vi "数据库更新.vi"(0 "设备号":string(combo)="01", 9 "数据":string[](array[string])=["123456", "ZHANG", "1", "1", "20150718", "20150719", "5", "Q14073-01", "100", "100", "100", "100", "200", "200", "200", "300", "300", "300", "300", "300", "300", "300", "300"], 11 "error in (no error)":errorcluster) -> (15 "error out":errorcluster)   [LabVIEW 2013]
panel:
  out "连接的字符串":string
  in  "数据名":string[](array[string])=["CZZ", "WC", "HG", "KSSJ", "JSSJ", "FGCS", "SBID", "Date1", "Date2", "Date3", "Date4", "Date5", "Date6", "Date7", "Date8", "Date9", "Date10", "Date11", "Date12", "Date13", "Date14", "Date15"]
  # "CZZ\nWC\nHG\nKSSJ\nJSSJ\nFGCS\nSBID\nDate1\nDate2\nDate3\nDate4\nDate5\nDate6\nDate7\nDate8\nDate9\nDate10\nDate11\nDate12\nDate13\nDate14\nDate15"
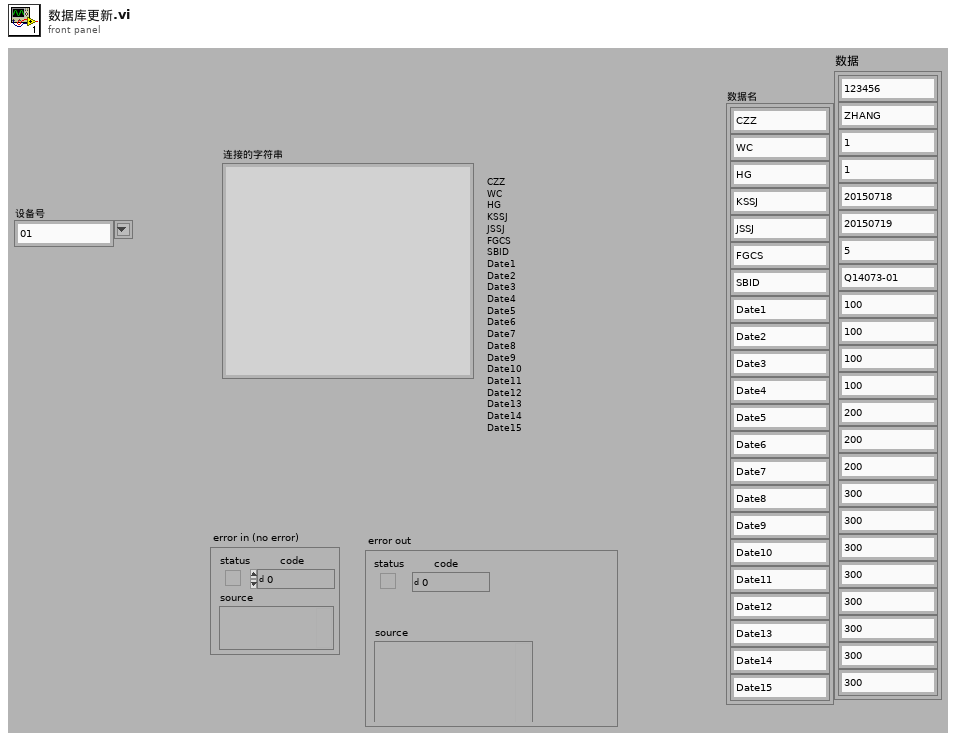
[diagram p1: front panel]
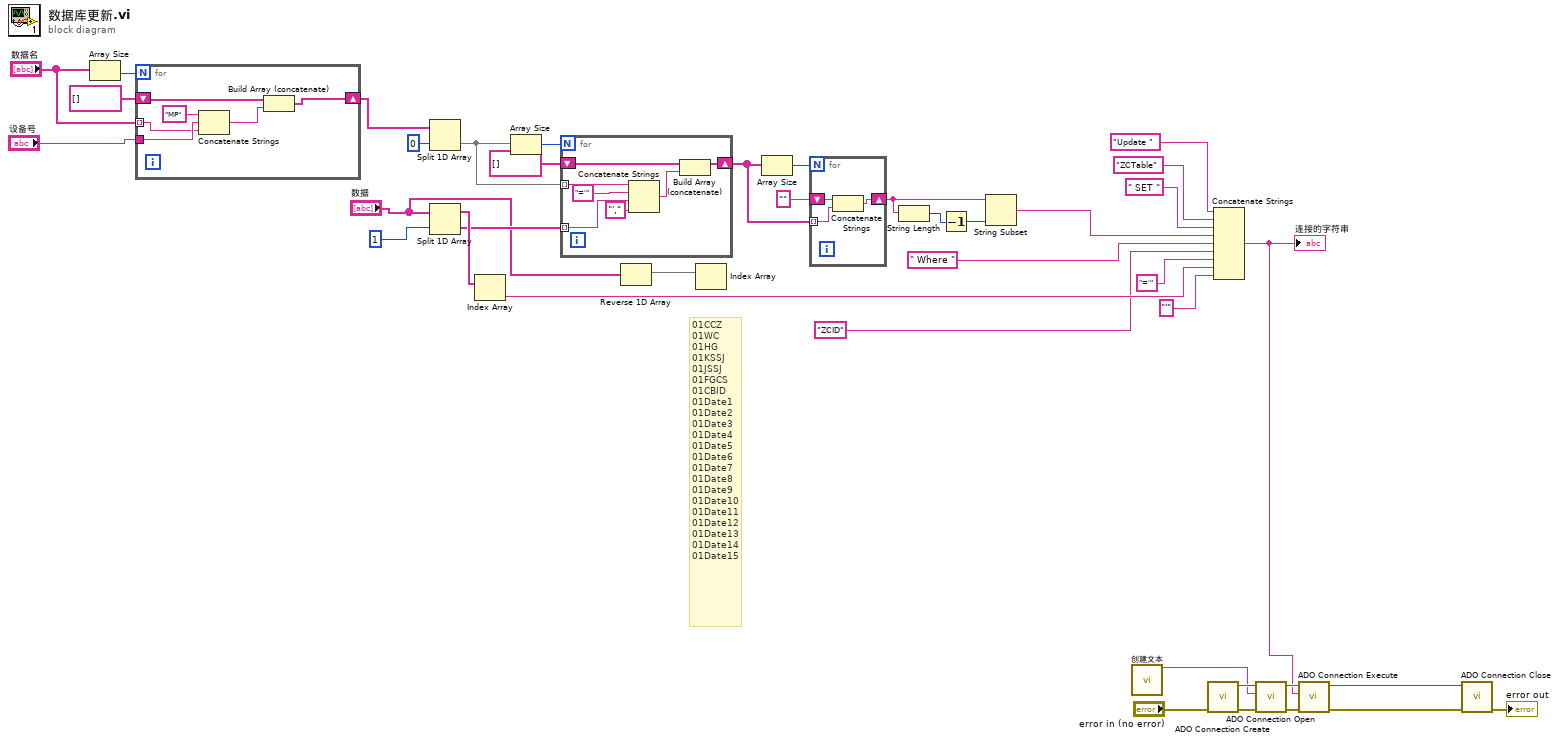
[diagram p0: block diagram]
diagram:
  # "01CCZ\n01WC\n01HG\n01KSSJ\n01JSSJ\n01FGCS\n01CBID\n01Date1\n01Date2\n01Date3\n01Date4\n01Date5\n01Date6\n01Date7\n01Date8\n01Date9\n01Date10\n01Date11\n01Date12\n01Date13\n01Date14\n01Date15"
  n1 = Array Size(array="数据名") -> (size(s)=w11:i32)
  n2 = for {
    N: w11 -> [_]
    tunnel: "数据名" -> [w41] mode=indexing
    shift-right: [w43] -> w7
    shift-left: string[] [] -> [w45]
    tunnel: "设备号" -> [w42]
    n3 = Concatenate Strings("MP" ("字符串"), w42, w41) -> (w44:string)
    n4 = Build Array (concatenate)(w45, w44) -> (w43:string[])
  }
  n5 = Split 1D Array(array=w7, index=0 ("索引")) -> (second subarray=w27:string[])  [unwired: 1 out]
  n6 = Split 1D Array(array="数据", index=1 ("索引列")) -> (first subarray=w29:string[], second subarray=w26:string[])
  n7 = Index Array(array=w29) -> (element=w14:string)  [unwired: 1 in]
  n8 = Array Size(array=w27) -> (size(s)=w28:i32)
  n9 = for {
    N: w28 -> [_]
    tunnel: w27 -> [w52] mode=indexing
    shift-right: [w49] -> w24
    shift-left: string[] [] -> [w48]
    tunnel: w26 -> [w47] mode=indexing
    n10 = Concatenate Strings(w52, "='" ("字符串"), w47, "'," ("字符串")) -> (w50:string)
    n11 = Build Array (concatenate)(w48, w50) -> (w49:string[])
  }
  n12 = Reverse 1D Array(array="数据") -> (reversed array=w6:string[])
  n13 = Index Array(array=w6) -> ()  [unwired: 1 in, 1 out]
  n14 = Array Size(array=w24) -> (size(s)=w25:i32)
  n15 = for {
    N: w25 -> [_]
    tunnel: w24 -> [w55] mode=indexing
    shift-right: [w54] -> w23
    shift-left: "" -> [w53]
    n16 = Concatenate Strings(w53, w55) -> (w54:string)
  }
  n17 = String Length(string=w23) -> (length=w4:i32)
  n18 = Decrement(x=w4) -> (x-1=w3:i32)
  n19 = String Subset(string=w23, length (rest)=w3) -> (substring=w2:string)  [unwired: 1 in]
  n20 = call "创建文本"() -> ("Result"=w31:string)  [unwired: 14 in, 1 out]
  n21 = call "ADO Connection Create.vi"("error in (no error)"="error in (no error)") -> ("error out"=w38:errorcluster, "ADODB._Connection Out"=w37:refnum<k7>)  [unwired: 9 out]
  n22 = Concatenate Strings("Update " ("字符串"), "ZCTable" ("数据库名"), " SET " ("字符串"), w2, " Where " ("字符串"), "ZCID" ("索引列名"), "='" ("字符串"), w14, "'" ("字符串")) -> (w5:string)
  "连接的字符串" <- w5
  n23 = call "ADO Connection Open.vi"("error in (no error)"=w38, "ConnectionString"=w31, "ADODB._Connection In"=w37) -> ("error out"=w36:errorcluster, "ADODB._Connection Out"=w35:refnum<k7>)  [unwired: 7 out]
  n24 = call "ADO Connection Execute.vi"("error in (no error)"=w36, "CommandText"=w5, "ADODB._Connection In"=w35) -> ("error out"=w34:errorcluster, "ADODB._Connection Out"=w33:refnum<k7>)  [unwired: 7 out]
  n25 = call "ADO Connection Close.vi"("error in (no error)"=w34, "ADODB._Connection In"=w33) -> ("error out"=→"error out":errorcluster)  [unwired: 9 out]
